vi "Switching Levels Logic.vi"(8 "error in (no error)":errorcluster, 10 "buttons":bool[](array[boolean]), 11 "Elevator in":refnum<class "Elevator.lvclass">) -> (0 "error out":errorcluster, 2 "Cargo/Hatch":T1=enum."C0, Cargo Ground", 3 "Elevator out":refnum<class "Elevator.lvclass">)   [LabVIEW 2018, in "Elevator.lvlib" / "Elevator.lvclass"]
doc: "This VI handles the state switiching logic for the elevator."
uses:
  Elevator.lvclass
  Controls/Elevator Position.ctl
  Elevator.lvclass/Elevator.ctl
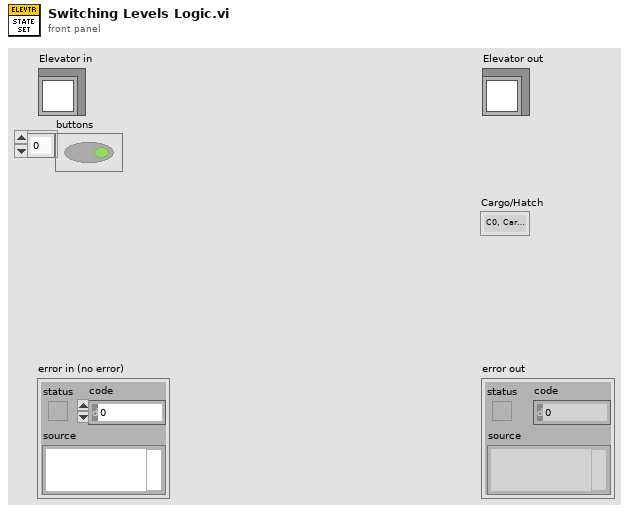
[diagram p1: front panel]
types:
  T1 = typedef "Elevator.lvlib/Elevator.lvclass/Elevator Position.ctl" = enum16{"CS, Cargo Ship Cargo", "C0, Cargo Ground", "C1, LV1 Cargo", "C2, LV2 Cargo", "C3, LV3 Cargo", "H0, LV1 Hatch", "H1, LV2 Hatch", "H2, LV3 Hatch"}
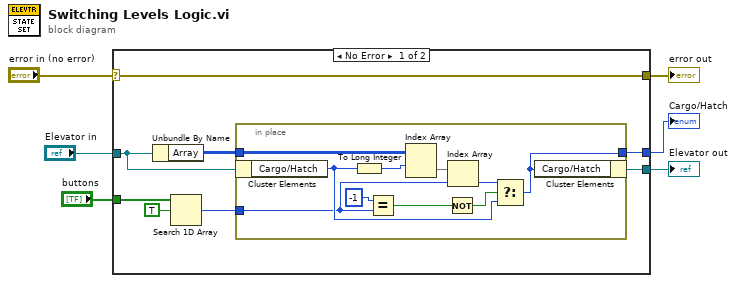
[diagram p0: block diagram]
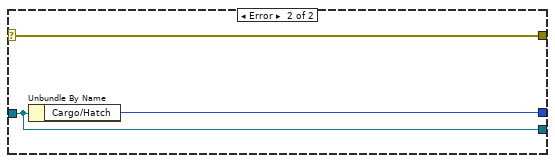
[diagram p2: hidden frame]
diagram:
  n1 = case shown="No Error" "error in (no error)" {
    selector: "error in (no error)" -> [w14 w27]
    tunnel: [w14 w27] -> w5
    tunnel: [w13 w26] -> w3
    tunnel: "Elevator in" -> [w8 w26]
    tunnel: [w12 w25] -> w2
    tunnel: "buttons" -> [w10 _]
    frame No Error {
      n2 = Unbundle By Name(w8) -> ("Array"=w7:T1[][])
      n3 = Search 1D Array(1D array=w10, element=TRUE) -> (index of element=w11:i32)  [unwired: 1 in]
      n4 = in-place {
        in-place-border: [w15] -> w12
        in-place-border: w11 -> [w16]
        in-place-border: w7 -> [w17]
        n5 = in-place-cluster #1(w8) -> ("Cargo/Hatch"=w20:T1)
        n6 = To Long Integer(number=w20) -> (32bit integer=w24:i32)
        n7 = Equal?(x=-1, y=w16) -> (x = y?=w21:bool)
        n8 = Index Array(array=w17, index (row)=w24) -> (element=w23:T1[])  [unwired: 1 in]
        n9 = Not(x=w21) -> (.not. x?=w18:bool)
        n10 = Index Array(array=w23, index=w16) -> (element=w19:T1)
        n11 = Select(t=w19, s=w18, f=w20) -> (s? t:f=w15:T1)
        n12 = in-place-cluster #1("Cargo/Hatch"=w15) -> (w13:refnum<class "Elevator.lvclass">)
      }
    }
    frame Error {
      n13 = Unbundle By Name(w26) -> ("Cargo/Hatch"=w25:T1)
    }
  }
  "error out" <- w5
  "Elevator out" <- w3
  "Cargo/Hatch" <- w2
